vi "NanoScan ActiveX Sample.LV2018.vi"() -> ()   [LabVIEW 2018]
panel:
  in  "NanoScan.INanoScan":refnum<k7>
  out "Boolean":bool
  out "Sampling Res 1":sgl caption="Sampling Res" format="%.2f"
  out "Gain1":u32
  out "Aperture 1":cluster{"Intensity":sgl[], "Position":sgl[]}(graph)
  out "Sampling Res 2":sgl caption="Sampling Res" format="%.2f"
  out "Gain2":u32
  out "Aperture 2":cluster{"Intensity":sgl[], "Position":sgl[]}(graph)
  out "ROIs Aperture1":bool[](array[boolean])
  in  "Aperture":i32(slide) scale=1.0..2.0
  out "ROIs Aperture 2":bool[](array[boolean])
  in  "Position":sgl[](array[numeric]) format="%.2f"
  in  "Intensity":sgl[](array[numeric]) format="%.2f"
  in  "Ellipticity":sgl format="%.2f"
  in  "Roughness":sgl format="%.2f"
  in  "Goodness":sgl format="%.2f"
  in  "Irradiance":sgl format="%.2f"
  in  "Peak":sgl format="%.2f"
  in  "Centroid Pos":sgl format="%.2f"
  in  "BeamWidth":sgl format="%.2f"
  in  "Gain":i32
  in  "Set Gain":bool
  in  "Row":i32
  out "Parameters Array":string[][](array[string])
  in  "ROIs Ap2":i16
  in  "ROIs AP1":i16
  out "Intensity":sgl[](array[numeric]) format="%.2f"
  out "Position":sgl[](array[numeric]) format="%.2f"
  in  "Apr Right":sgl format="%.2f"
  in  "AprLeft":sgl format="%.2f"
  out "Parameters":i32[](listbox)
  in  "Filter":sgl=2.0 min=2 max=190 step=1 format="%.2f"
  in  "Set Filter":bool
  out "DAQ ON?":bool
  in  "Auto Find":bool
  in  "DAQ":bool caption="stop"
  in  "Exit":bool
  in  "13.5% Width":bool
  in  "Irradiance":bool
  in  "4Sigma Width":bool
  in  "Peak Pos":bool
  in  "50% Width":bool
  in  "Centroid Pos":bool
  in  "Peak Separation":bool caption="4Sigma Width 5"
  in  "Centroid Separation":bool
  in  "Gaussian Fit":bool
  in  "Ellipticity":bool
  in  "Select Sampling":sgl=0.09 min=0.0057 step=0.01 format="%.4f"
  in  "Set Sampling":bool
  out "Gains":u32[](array[numeric])
  in  "Select Rotation Rate":u16(ring) items=["1.25", "2.50", "5.00", "10.00", "20.00"]
  out "Measured Rotation [Hz]":sgl(knob) scale=1.25..20.0 scale format="%.2f"
  in  "Set Rotation":bool
  in  "Speed":sgl format="%.2f"
  in  "Gains 2":variant[](array[variant])
  out "pvarHeadInfo":variant
  in  "Speeds 2":variant[](array[variant])
  out "error out":errorcluster
  out "Speeds":sgl[](array[numeric]) format="%.2f"
  # "NanoScan"
  # "Parameters"
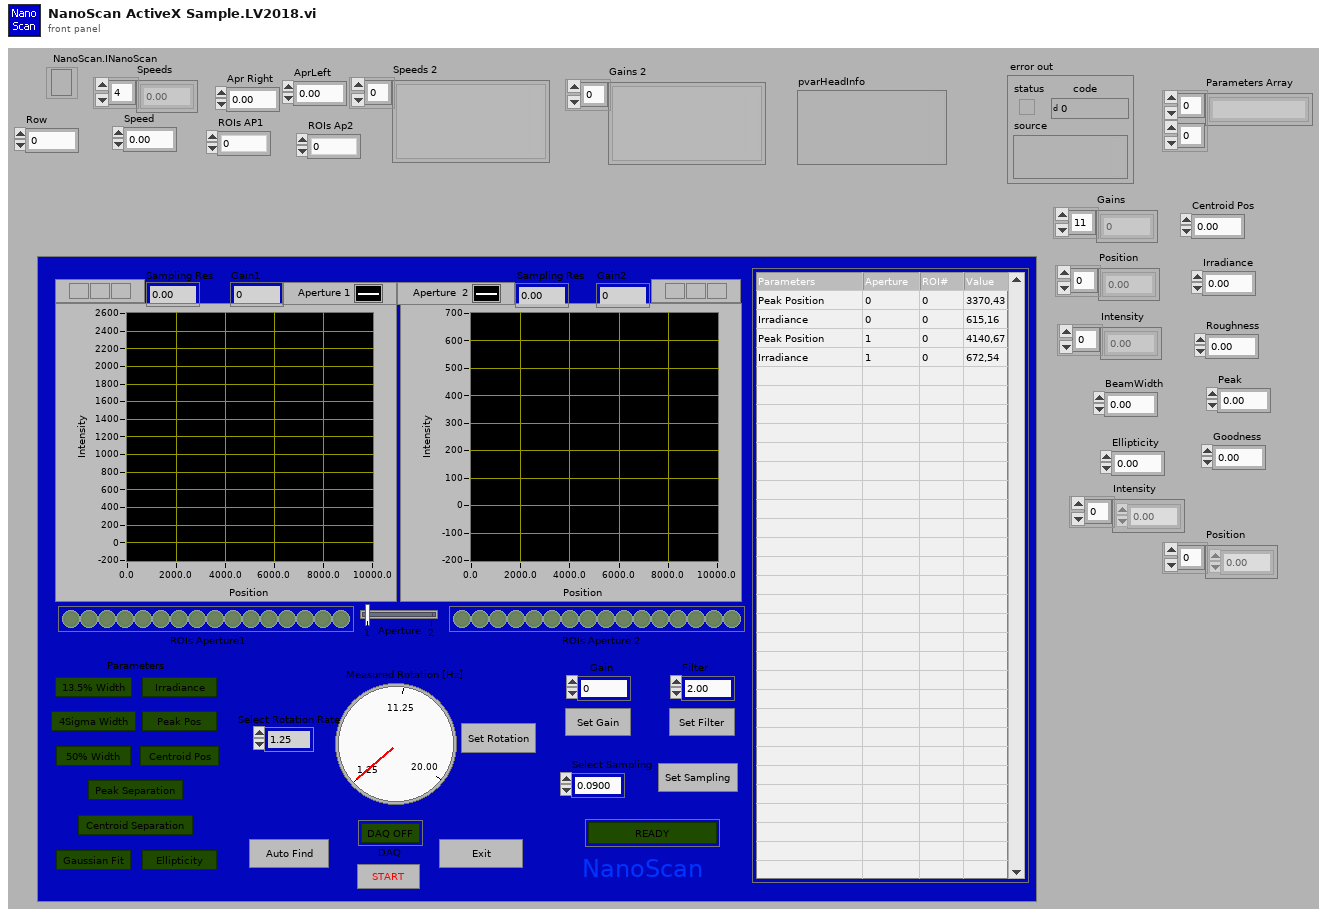
[diagram p1: front panel]
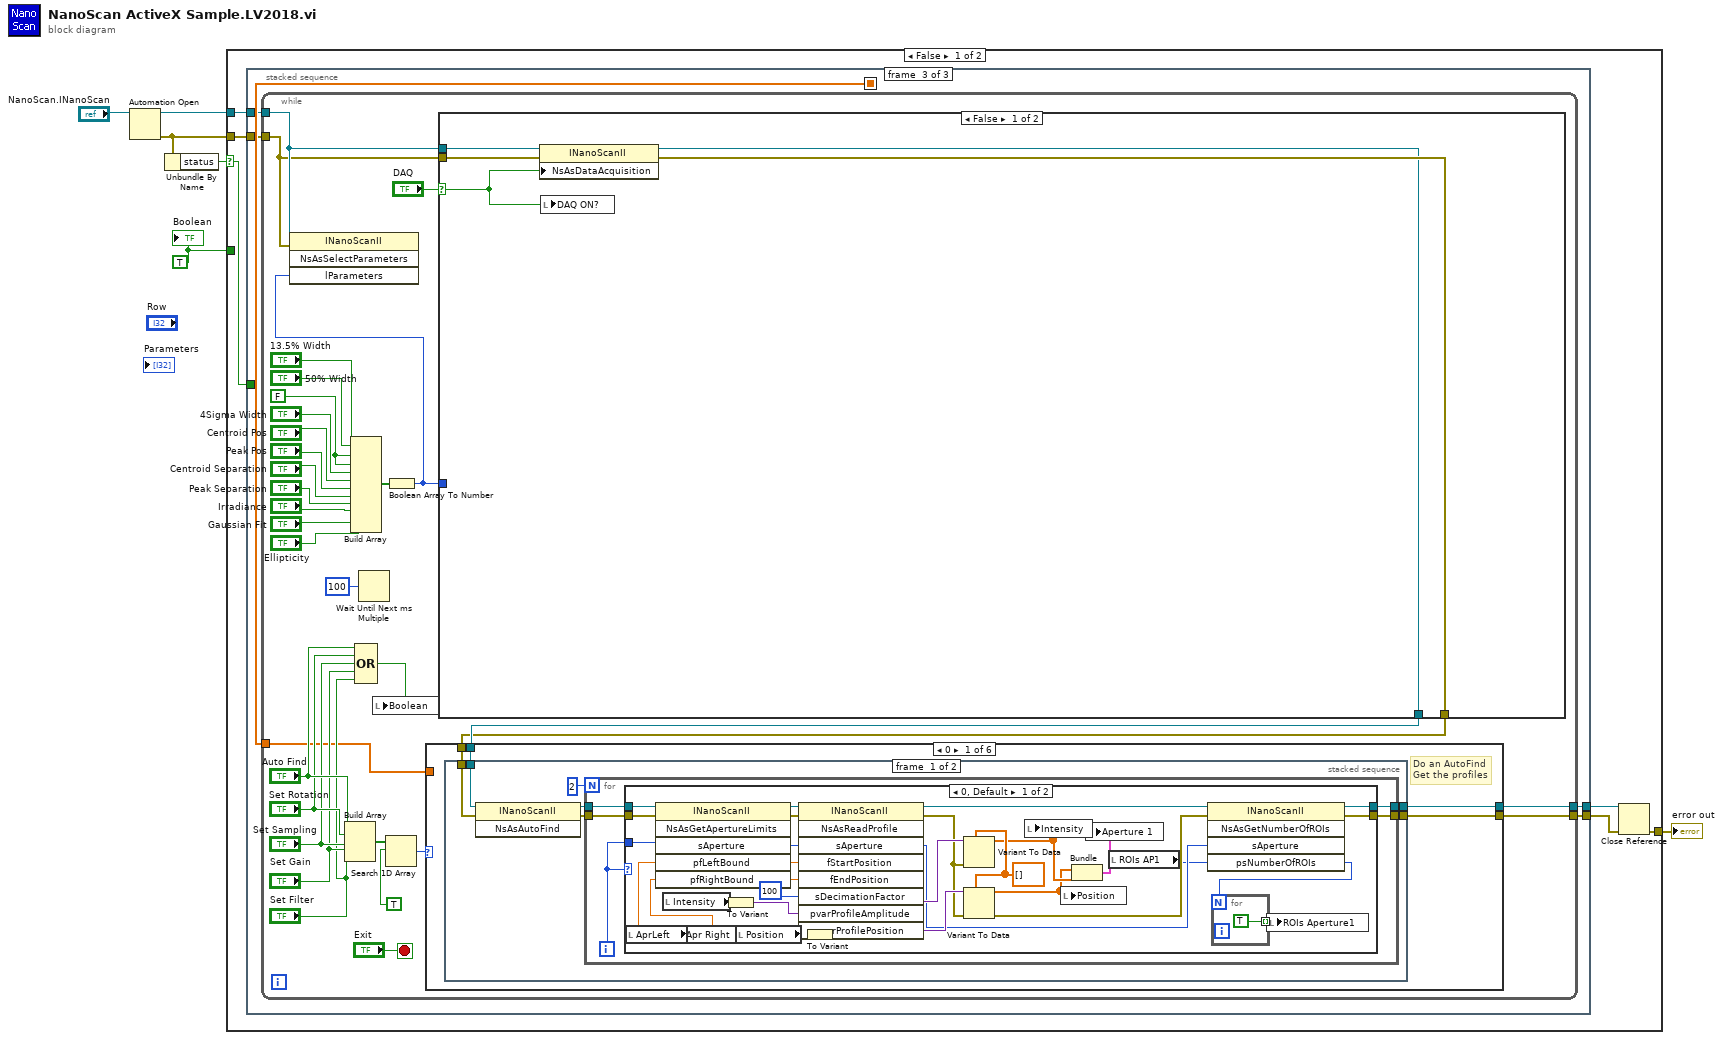
[diagram p0: block diagram]
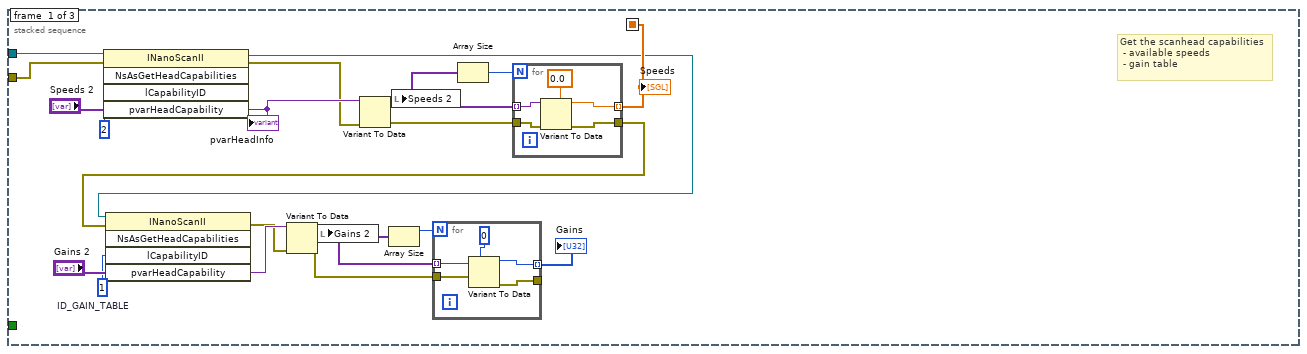
[diagram p2: hidden frame]
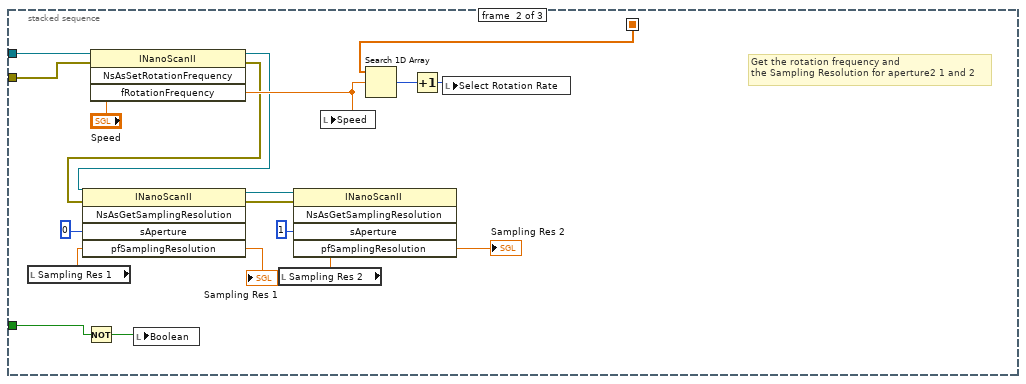
[diagram p3: hidden frame]
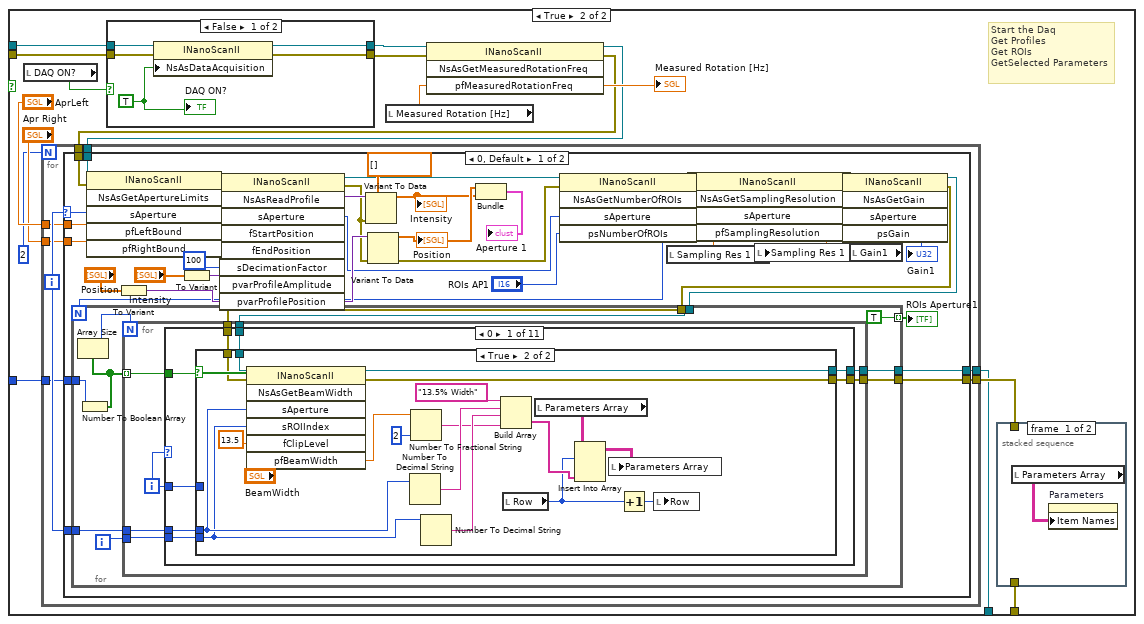
[diagram p4: hidden frame]
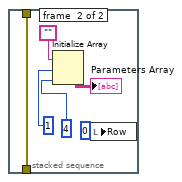
[diagram p5: hidden frame]
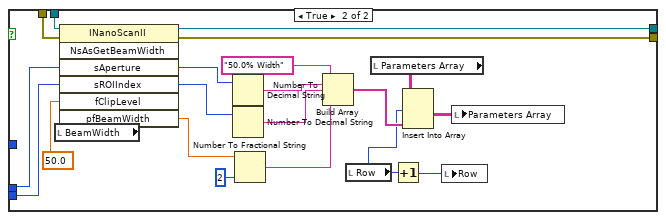
[diagram p8: hidden frame]
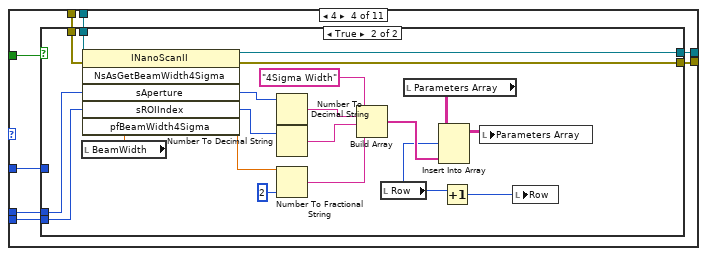
[diagram p10: hidden frame]
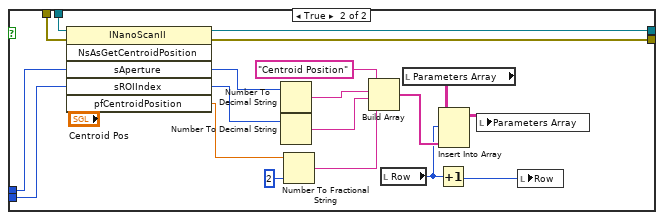
[diagram p13: hidden frame]
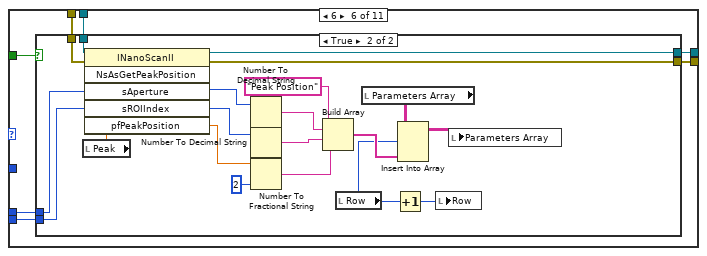
[diagram p14: hidden frame]
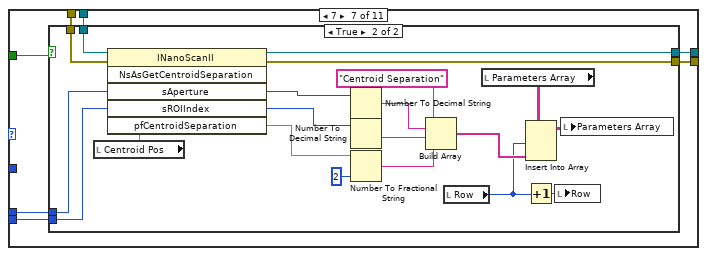
[diagram p16: hidden frame]
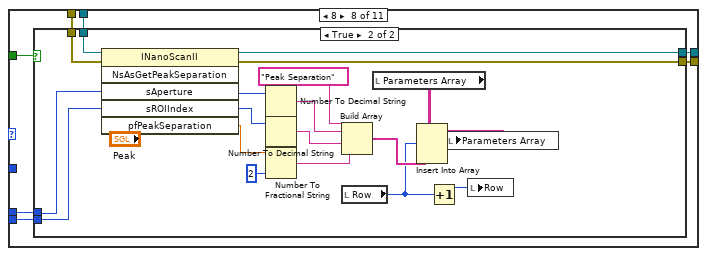
[diagram p18: hidden frame]
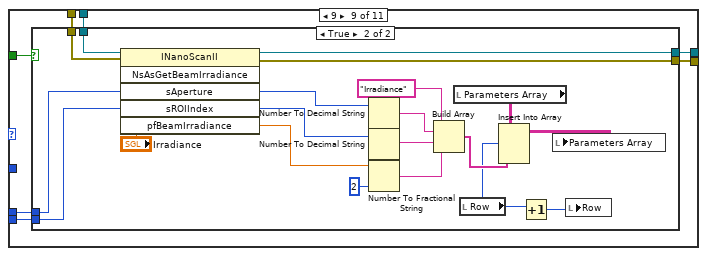
[diagram p20: hidden frame]
diagram:
  w1 = TRUE
  n1 = Automation Open(Automation Refnum="NanoScan.INanoScan") -> (Automation Refnum=w3:refnum<k7>, error out=w4:errorcluster)  [unwired: 1 in, 2 out]
  n2 = Unbundle By Name(w4) -> ("status"=w5:bool)
  n3 = case shown="False" w5 {
    selector: w5 -> [w12 w1002]
    tunnel: w4 -> [w11 w1000]
    tunnel: w3 -> [w10 w999]
    tunnel: [w7 w1000] -> w2
    tunnel: w1 -> [_ _]
    frame False {
      n4 = stacked-sequence {
        seq-local: [w27 _ _] -> [_ w61 w66]
        tunnel: w12 -> [_ w58 _]
        tunnel: w11 -> [w23 w43 w65]
        tunnel: w10 -> [w24 w56 w64]
        tunnel: [_ _ w63] -> w9
        tunnel: [_ _ w62] -> w8
        frame #0 {
          w17 = 1  # ID_GAIN_TABLE
          # "Get the scanhead capabilities\n - available speeds\n - gain table"
          n5 = invoke class="INanoScanII" method="NsAsGetHeadCapabilities"(reference=w24, error in=w23, "lCapabilityID"=2, "pvarHeadCapability"="Speeds 2") -> (reference out=w16:refnum<k7>, error out=w19:errorcluster, "pvarHeadCapability"=w22:variant)  [unwired: 1 in, 2 out]
          "pvarHeadInfo" <- w22
          n6 = Variant To Data(error in=w19, Variant=w22) -> (data=w26:variant[], error out=w28:errorcluster)  [unwired: 1 in]
          n7 = local write "Speeds 2"(w26) -> ()
          n8 = Array Size(array=w26) -> (size(s)=w25:i32)
          n9 = for {
            N: w25 -> [_]
            tunnel: w26 -> [w37] mode=indexing
            tunnel: [w36] -> w27 mode=indexing
            tunnel: w28 -> [w35]
            tunnel: [w33] -> w15
            n10 = Variant To Data(error in=w35, type=sgl 0.0, Variant=w37) -> (data=w36:sgl, error out=w33:errorcluster)
          }
          "Speeds" <- w27
          n11 = invoke class="INanoScanII" method="NsAsGetHeadCapabilities"(reference=w16, error in=w15, "lCapabilityID"=w17, "pvarHeadCapability"="Gains 2") -> (error out=w13:errorcluster, "pvarHeadCapability"=w14:variant)  [unwired: 1 in, 3 out]
          n12 = Variant To Data(error in=w13, Variant=w14) -> (data=w29:variant[], error out=w30:errorcluster)  [unwired: 1 in]
          n13 = local write "Gains 2"(w29) -> ()
          n14 = Array Size(array=w29) -> (size(s)=w31:i32)
          n15 = for {
            N: w31 -> [_]
            tunnel: w29 -> [w41] mode=indexing
            tunnel: w30 -> [w40]
            tunnel: [w39] -> w32 mode=indexing
            tunnel: [w38] -> _
            n16 = Variant To Data(error in=w40, type=u32 0, Variant=w41) -> (data=w39:u32, error out=w38:errorcluster)
          }
          "Gains" <- w32
        }
        frame #1 {
          # "Get the rotation frequency and\nthe Sampling Resolution for aperture2 1 and 2"
          n17 = local read "Sampling Res 1"() -> (w46:sgl)
          n18 = Not(x=w58) -> (.not. x?=w57:bool)
          n19 = invoke class="INanoScanII" method="NsAsSetRotationFrequency"(reference=w56, error in=w43, "fRotationFrequency"="Speed") -> (reference out=w53:refnum<k7>, error out=w52:errorcluster, "fRotationFrequency"=w55:sgl)  [unwired: 1 in, 1 out]
          n20 = invoke class="INanoScanII" method="NsAsGetSamplingResolution"(reference=w53, error in=w52, "sAperture"=i16 0, "pfSamplingResolution"=w46) -> (reference out=w50:refnum<k7>, error out=w49:errorcluster, "pfSamplingResolution"=→"Sampling Res 1":sgl)  [unwired: 1 in, 2 out]
          n21 = local write "Boolean"(w57) -> ()
          n22 = local read "Sampling Res 2"() -> (w48:sgl)
          n23 = invoke class="INanoScanII" method="NsAsGetSamplingResolution"(reference=w50, error in=w49, "sAperture"=i16 1, "pfSamplingResolution"=w48) -> ("pfSamplingResolution"=→"Sampling Res 2":sgl)  [unwired: 1 in, 4 out]
          n24 = local write "Speed"(w55) -> ()
          n25 = Search 1D Array(1D array=w61, element=w55) -> (index of element=w60:i32)  [unwired: 1 out]
          n26 = Increment(x=w60) -> (x+1=w59:i32)
          n27 = local write "Select Rotation Rate"(w59) -> ()
        }
        frame #2 {
          n28 = while {
            tunnel: w66 -> [w72]
            tunnel: w65 -> [w73]
            tunnel: w64 -> [w74]
            tunnel: [w69] -> w63
            tunnel: [w68] -> w62
            stop <- "Exit" stop-if-true
            w91 = FALSE
            n29 = Build Array("Auto Find", "Set Rotation", "Set Sampling", "Set Gain", "Set Filter") -> (w97:bool[])
            n30 = Build Array("13.5% Width", "50% Width", w91, w91, "4Sigma Width", "Centroid Pos", "Peak Pos", "Centroid Separation", "Peak Separation", "Irradiance", "Gaussian Fit", "Ellipticity") -> (w82:bool[])
            n31 = Compound Arithmetic op=OR("Auto Find", "Set Rotation", "Set Sampling", "Set Gain", "Set Filter") -> (w76:bool)
            n32 = Wait Until Next ms Multiple(millisecond multiple=u32 100) -> ()  [unwired: 1 out]
            n33 = local write "Boolean"(w76) -> ()
            n34 = Search 1D Array(1D array=w97, element=TRUE) -> (index of element=w95:i32)  [unwired: 1 out]
            n35 = Boolean Array To Number(Boolean array=w82) -> (number=w67:u32)
            n36 = invoke class="INanoScanII" method="NsAsSelectParameters"(reference=w74, error in=w73, "lParameters"=w67) -> ()  [unwired: 1 in, 4 out]
            n37 = case shown="False" "DAQ" {
              selector: "DAQ" -> [w99 _]
              tunnel: w67 -> [_ w115]
              tunnel: w74 -> [w103 w114]
              tunnel: w73 -> [w102 w113]
              tunnel: [w100 w105] -> w71
              tunnel: [w101 w104] -> w70
              frame False {
                n38 = property class="INanoScanII"(reference=w103, error in=w102, "NsAsDataAcquisition"=w99) -> (reference out=w100:refnum<k7>, error out=w101:errorcluster)
                n39 = local write "DAQ ON?"(w99) -> ()
              }
              frame True {
                # "Start the Daq\nGet Profiles\nGet ROIs\nGetSelected Parameters"
                n40 = local read "DAQ ON?"() -> (w119:bool)
                n41 = case shown="False" w119 {
                  tunnel: w114 -> [w866 w868]
                  tunnel: w113 -> [w864 w867]
                  tunnel: [w865 w868] -> w112
                  tunnel: [w863 w867] -> w111
                  frame False {
                    w862 = TRUE ("NsAsDataAcquisition")
                    n42 = property class="INanoScanII"(reference=w866, error in=w864, "NsAsDataAcquisition"=w862) -> (reference out=w865:refnum<k7>, error out=w863:errorcluster)
                    "DAQ ON?" <- w862
                  }
                  frame True {
                  }
                }
                n43 = local read "Measured Rotation [Hz]"() -> (w110:sgl)
                n44 = invoke class="INanoScanII" method="NsAsGetMeasuredRotationFreq"(reference=w112, error in=w111, "pfMeasuredRotationFreq"=w110) -> (reference out=w108:refnum<k7>, error out=w107:errorcluster, "pfMeasuredRotationFreq"=→"Measured Rotation [Hz]":sgl)  [unwired: 1 in, 1 out]
                n45 = for {
                  N: i16 2 ("sAperture") -> [_]
                  tunnel: "AprLeft" -> [w133]
                  tunnel: "Apr Right" -> [w132]
                  tunnel: w115 -> [w131]
                  tunnel: w108 -> [w130]
                  tunnel: w107 -> [w129]
                  tunnel: [w128] -> w105
                  tunnel: [w127] -> w106
                  i -> [w134]
                  n46 = case shown="0, Default" w134 {
                    selector: w134 -> [w166 w535]
                    tunnel: w133 -> [w168 w537]
                    tunnel: w132 -> [w167 w536]
                    tunnel: w131 -> [w178 w541]
                    tunnel: w134 -> [w177 w540]
                    tunnel: w130 -> [w170 w539]
                    tunnel: w129 -> [w169 w538]
                    tunnel: [w138 w509] -> w128
                    tunnel: [w137 w508] -> w127
                    frame 0, Default {
                      n47 = invoke class="INanoScanII" method="NsAsGetApertureLimits"(reference=w170, error in=w169, "sAperture"=w166, "pfLeftBound"=w168, "pfRightBound"=w167) -> (reference out=w165:refnum<k7>, error out=w164:errorcluster, "sAperture"=w163:i16, "pfLeftBound"=w159:sgl, "pfRightBound"=w158:sgl)  [unwired: 1 in, 1 out]
                      n48 = To Variant(anything="Position") -> (Variant=w160:variant)
                      n49 = To Variant(anything="Intensity") -> (Variant=w162:variant)
                      n50 = invoke class="INanoScanII" method="NsAsReadProfile"(reference=w165, error in=w164, "sAperture"=w163, "fStartPosition"=w159, "fEndPosition"=w158, "sDecimationFactor"=i16 100, "pvarProfileAmplitude"=w162, "pvarProfilePosition"=w160) -> (reference out=w154:refnum<k7>, error out=w155:errorcluster, "sAperture"=w152:i16, "pvarProfileAmplitude"=w157:variant, "pvarProfilePosition"=w156:variant)  [unwired: 1 in, 4 out]
                      n51 = Variant To Data(error in=w155, type=sgl[] [] ("Intensity"), Variant=w157) -> (data=w171:sgl[])  [unwired: 1 out]
                      "Intensity" <- w171
                      n52 = Variant To Data(error in=w155, Variant=w156) -> (data=w172:sgl[], error out=w153:errorcluster)  [unwired: 1 in]
                      "Position" <- w172
                      n53 = Bundle("Position"=w172, "Intensity"=w171) -> (→"Aperture 1":cluster{"Position":sgl[], "Intensity":sgl[]})  [unwired: 1 out]
                      n54 = invoke class="INanoScanII" method="NsAsGetNumberOfROIs"(reference=w154, error in=w153, "sAperture"=w152, "psNumberOfROIs"="ROIs AP1") -> (reference out=w150:refnum<k7>, error out=w149:errorcluster, "sAperture"=w148:i16, "psNumberOfROIs"=w142:i16)  [unwired: 1 in, 1 out]
                      n55 = local read "Sampling Res 1"() -> (w143:sgl)
                      n56 = invoke class="INanoScanII" method="NsAsGetSamplingResolution"(reference=w150, error in=w149, "sAperture"=w148, "pfSamplingResolution"=w143) -> (reference out=w147:refnum<k7>, error out=w146:errorcluster, "sAperture"=w145:i16, "pfSamplingResolution"=w144:sgl)  [unwired: 1 in, 1 out]
                      n57 = local write "Sampling Res 1"(w144) -> ()
                      n58 = local read "Gain1"() -> (w136:u32)
                      n59 = invoke class="INanoScanII" method="NsAsGetGain"(reference=w147, error in=w146, "sAperture"=w145, "psGain"=w136) -> (reference out=w139:refnum<k7>, error out=w140:errorcluster, "psGain"=→"Gain1":i16)  [unwired: 1 in, 2 out]
                      n60 = for {
                        N: w142 -> [_]
                        tunnel: w178 -> [w188]
                        tunnel: w177 -> [w185]
                        tunnel: [TRUE] -> w141 mode=indexing
                        tunnel: w140 -> [w183]
                        tunnel: w139 -> [w182]
                        tunnel: [w181] -> w138
                        tunnel: [w180] -> w137
                        i -> [w179]
                        n61 = Number To Boolean Array(number=w188) -> (Boolean array=w186:bool[])
                        n62 = Array Size(array=w186) -> (size(s)=w187:i32)
                        n63 = for {
                          N: w187 -> [_]
                          tunnel: w186 -> [w193] mode=indexing
                          tunnel: w185 -> [w196]
                          tunnel: w179 -> [w195]
                          tunnel: w183 -> [w192]
                          tunnel: w182 -> [w191]
                          tunnel: [w190] -> w181
                          tunnel: [w189] -> w180
                          i -> [w194]
                          n64 = case shown="0" w194 {
                            tunnel: w193 -> [w204 w233 _ w264 w295 w324 w353 w380 w411 w440 w477]
                            tunnel: w196 -> [w203 w231 _ w265 w291 w323 w352 w382 w410 w439 w476]
                            tunnel: w195 -> [w202 w226 _ w263 w290 w322 w351 w381 w409 w438 w475]
                            tunnel: w194 -> [w201 w232 _ w266 _ _ _ _ _ _ _]
                            tunnel: w192 -> [w200 w229 w257 w261 w289 w319 w349 w378 w407 w434 w471]
                            tunnel: w191 -> [w199 w230 w258 w262 w294 w318 w350 w379 w408 w435 w472]
                            tunnel: [w198 w227 w258 w260 w293 w321 w348 w377 w406 w437 w474] -> w190
                            tunnel: [w197 w228 w257 w259 w292 w320 w347 w376 w405 w436 w473] -> w189
                            frame 0 {
                              n65 = case shown="True" w204 {
                                tunnel: w203 -> [_ w210]
                                tunnel: w202 -> [_ w209]
                                tunnel: w201 -> [_ _]
                                tunnel: w200 -> [w205 w215]
                                tunnel: w199 -> [w206 w214]
                                tunnel: [w206 w213] -> w198
                                tunnel: [w205 w212] -> w197
                                frame False {
                                }
                                frame True {
                                n66 = invoke class="INanoScanII" method="NsAsGetBeamWidth"(reference=w214, error in=w215, "sAperture"=w210, "sROIIndex"=w209, "fClipLevel"=13.5, "pfBeamWidth"="BeamWidth") -> (reference out=w213:refnum<k7>, error out=w212:errorcluster, "pfBeamWidth"=w207:sgl)  [unwired: 1 in, 4 out]
                                n67 = Number To Decimal String(number=w210) -> (decimal integer string=w224:string)  [unwired: 1 out]
                                n68 = Number To Fractional String(number=w207, precision (6)=i16 2) -> (F-format string=w222:string)  [unwired: 2 out]
                                n69 = Number To Decimal String(number=w209) -> (decimal integer string=w223:string)  [unwired: 1 out]
                                n70 = Build Array("13.5% Width", w224, w223, w222) -> (w221:string[])
                                n71 = local read "Row"() -> (w217:i32)
                                n72 = local read "Parameters Array"() -> (w219:string[][])
                                n73 = Insert Into Array(array=w219, index (row)=w217, new element=w221) -> (w218:string[][])  [unwired: 1 in]
                                n74 = local write "Parameters Array"(w218) -> ()
                                n75 = Increment(x=w217) -> (x+1=w220:i32)
                                n76 = local write "Row"(w220) -> ()
                                }
                              }
                            }
                            frame 1 {
                              n77 = case shown="False" w233 {
                                tunnel: w232 -> [_ _]
                                tunnel: w231 -> [_ w244]
                                tunnel: w230 -> [w234 w246]
                                tunnel: w229 -> [w235 w245]
                                tunnel: [w235 w236] -> w228
                                tunnel: [w234 w238] -> w227
                                tunnel: w226 -> [_ w243]
                                frame False {
                                }
                                frame True {
                                n78 = local read "BeamWidth"() -> (w241:sgl)
                                n79 = invoke class="INanoScanII" method="NsAsGetBeamWidth"(reference=w246, error in=w245, "sAperture"=w244, "sROIIndex"=w243, "fClipLevel"=sgl 50.0, "pfBeamWidth"=w241) -> (reference out=w238:refnum<k7>, error out=w236:errorcluster, "sAperture"=w237:i16, "sROIIndex"=w240:i16, "pfBeamWidth"=w239:sgl)  [unwired: 1 in, 2 out]
                                n80 = Number To Decimal String(number=w237) -> (decimal integer string=w255:string)  [unwired: 1 out]
                                n81 = Number To Decimal String(number=w240) -> (decimal integer string=w254:string)  [unwired: 1 out]
                                n82 = Number To Fractional String(number=w239, precision (6)=i16 2) -> (F-format string=w253:string)  [unwired: 2 out]
                                n83 = Build Array("50.0% Width", w255, w254, w253) -> (w251:string[])
                                n84 = local read "Row"() -> (w249:i32)
                                n85 = local read "Parameters Array"() -> (w252:string[][])
                                n86 = Increment(x=w249) -> (x+1=w248:i32)
                                n87 = Insert Into Array(array=w252, index (row)=w249, new element=w251) -> (w250:string[][])  [unwired: 1 in]
                                n88 = local write "Row"(w248) -> ()
                                n89 = local write "Parameters Array"(w250) -> ()
                                }
                              }
                            }
                            frame Default {
                            }
                            frame 4 {
                              n90 = case shown="True" w264 {
                                tunnel: w266 -> [_ _]
                                tunnel: w265 -> [_ w273]
                                tunnel: w263 -> [_ w272]
                                tunnel: w262 -> [w268 w278]
                                tunnel: w261 -> [w267 w277]
                                tunnel: [w268 w276] -> w260
                                tunnel: [w267 w275] -> w259
                                frame False {
                                }
                                frame True {
                                n91 = local read "BeamWidth"() -> (w274:sgl)
                                n92 = invoke class="INanoScanII" method="NsAsGetBeamWidth4Sigma"(reference=w278, error in=w277, "sAperture"=w273, "sROIIndex"=w272, "pfBeamWidth4Sigma"=w274) -> (reference out=w276:refnum<k7>, error out=w275:errorcluster, "sAperture"=w271:i16, "sROIIndex"=w270:i16, "pfBeamWidth4Sigma"=w269:sgl)  [unwired: 1 in, 1 out]
                                n93 = Number To Decimal String(number=w271) -> (decimal integer string=w287:string)  [unwired: 1 out]
                                n94 = Number To Decimal String(number=w270) -> (decimal integer string=w286:string)  [unwired: 1 out]
                                n95 = Number To Fractional String(number=w269, precision (6)=i16 2) -> (F-format string=w285:string)  [unwired: 2 out]
                                n96 = Build Array("4Sigma Width", w287, w286, w285) -> (w284:string[])
                                n97 = local read "Row"() -> (w281:i32)
                                n98 = local read "Parameters Array"() -> (w282:string[][])
                                n99 = Insert Into Array(array=w282, index (row)=w281, new element=w284) -> (w283:string[][])  [unwired: 1 in]
                                n100 = Increment(x=w281) -> (x+1=w280:i32)
                                n101 = local write "Parameters Array"(w283) -> ()
                                n102 = local write "Row"(w280) -> ()
                                }
                              }
                            }
                            frame 5 {
                              n103 = case shown="False" w295 {
                                tunnel: w294 -> [w296 w307]
                                tunnel: [w296 w306] -> w293
                                tunnel: [w297 w305] -> w292
                                tunnel: w291 -> [_ w303]
                                tunnel: w290 -> [_ w302]
                                tunnel: w289 -> [w297 w298]
                                frame False {
                                }
                                frame True {
                                n104 = invoke class="INanoScanII" method="NsAsGetCentroidPosition"(reference=w307, error in=w298, "sAperture"=w303, "sROIIndex"=w302, "pfCentroidPosition"="Centroid Pos") -> (reference out=w306:refnum<k7>, error out=w305:errorcluster, "sAperture"=w301:i16, "sROIIndex"=w300:i16, "pfCentroidPosition"=w299:sgl)  [unwired: 1 in, 1 out]
                                n105 = Number To Decimal String(number=w301) -> (decimal integer string=w316:string)  [unwired: 1 out]
                                n106 = Number To Decimal String(number=w300) -> (decimal integer string=w315:string)  [unwired: 1 out]
                                n107 = Number To Fractional String(number=w299, precision (6)=i16 2) -> (F-format string=w314:string)  [unwired: 2 out]
                                n108 = Build Array("Centroid Position", w316, w315, w314) -> (w313:string[])
                                n109 = local read "Row"() -> (w309:i32)
                                n110 = local read "Parameters Array"() -> (w312:string[][])
                                n111 = Increment(x=w309) -> (x+1=w310:i32)
                                n112 = Insert Into Array(array=w312, index (row)=w309, new element=w313) -> (w311:string[][])  [unwired: 1 in]
                                n113 = local write "Parameters Array"(w311) -> ()
                                n114 = local write "Row"(w310) -> ()
                                }
                              }
                            }
                            frame 6 {
                              n115 = case shown="True" w324 {
                                tunnel: w323 -> [_ w331]
                                tunnel: w322 -> [_ w330]
                                tunnel: [w326 w336] -> w321
                                tunnel: [w325 w335] -> w320
                                tunnel: w319 -> [w325 w334]
                                tunnel: w318 -> [w326 w333]
                                frame False {
                                }
                                frame True {
                                n116 = local read "Peak"() -> (w332:sgl)
                                n117 = invoke class="INanoScanII" method="NsAsGetPeakPosition"(reference=w333, error in=w334, "sAperture"=w331, "sROIIndex"=w330, "pfPeakPosition"=w332) -> (reference out=w336:refnum<k7>, error out=w335:errorcluster, "sAperture"=w329:i16, "sROIIndex"=w328:i16, "pfPeakPosition"=w327:sgl)  [unwired: 1 in, 1 out]
                                n118 = Number To Decimal String(number=w329) -> (decimal integer string=w345:string)  [unwired: 1 out]
                                n119 = Number To Decimal String(number=w328) -> (decimal integer string=w344:string)  [unwired: 1 out]
                                n120 = Number To Fractional String(number=w327, precision (6)=i16 2) -> (F-format string=w343:string)  [unwired: 2 out]
                                n121 = Build Array("Peak Position", w345, w344, w343) -> (w342:string[])
                                n122 = local read "Row"() -> (w339:i32)
                                n123 = local read "Parameters Array"() -> (w340:string[][])
                                n124 = Increment(x=w339) -> (x+1=w338:i32)
                                n125 = Insert Into Array(array=w340, index (row)=w339, new element=w342) -> (w341:string[][])  [unwired: 1 in]
                                n126 = local write "Row"(w338) -> ()
                                n127 = local write "Parameters Array"(w341) -> ()
                                }
                              }
                            }
                            frame 7 {
                              n128 = case shown="True" w353 {
                                tunnel: w352 -> [_ w362]
                                tunnel: w351 -> [_ w361]
                                tunnel: w350 -> [w355 w364]
                                tunnel: w349 -> [w354 w363]
                                tunnel: [w355 w360] -> w348
                                tunnel: [w354 w359] -> w347
                                frame False {
                                }
                                frame True {
                                n129 = local read "Centroid Pos"() -> (w365:sgl)
                                n130 = invoke class="INanoScanII" method="NsAsGetCentroidSeparation"(reference=w364, error in=w363, "sAperture"=w362, "sROIIndex"=w361, "pfCentroidSeparation"=w365) -> (reference out=w360:refnum<k7>, error out=w359:errorcluster, "sAperture"=w358:i16, "sROIIndex"=w357:i16, "pfCentroidSeparation"=w356:sgl)  [unwired: 1 in, 1 out]
                                n131 = Number To Decimal String(number=w358) -> (decimal integer string=w374:string)  [unwired: 1 out]
                                n132 = Number To Decimal String(number=w357) -> (decimal integer string=w373:string)  [unwired: 1 out]
                                n133 = Number To Fractional String(number=w356, precision (6)=i16 2) -> (F-format string=w372:string)  [unwired: 2 out]
                                n134 = Build Array("Centroid Separation", w374, w373, w372) -> (w369:string[])
                                n135 = local read "Row"() -> (w368:i32)
                                n136 = local read "Parameters Array"() -> (w371:string[][])
                                n137 = Insert Into Array(array=w371, index (row)=w368, new element=w369) -> (w370:string[][])  [unwired: 1 in]
                                n138 = Increment(x=w368) -> (x+1=w367:i32)
                                n139 = local write "Row"(w367) -> ()
                                n140 = local write "Parameters Array"(w370) -> ()
                                }
                              }
                            }
                            frame 8 {
                              n141 = case shown="True" w380 {
                                tunnel: w382 -> [_ w386]
                                tunnel: w381 -> [_ w385]
                                tunnel: w379 -> [w384 w394]
                                tunnel: w378 -> [w383 w393]
                                tunnel: [w384 w392] -> w377
                                tunnel: [w383 w391] -> w376
                                frame False {
                                }
                                frame True {
                                n142 = invoke class="INanoScanII" method="NsAsGetPeakSeparation"(reference=w394, error in=w393, "sAperture"=w386, "sROIIndex"=w385, "pfPeakSeparation"="Peak") -> (reference out=w392:refnum<k7>, error out=w391:errorcluster, "sAperture"=w390:i16, "sROIIndex"=w389:i16, "pfPeakSeparation"=w388:sgl)  [unwired: 1 in, 1 out]
                                n143 = Number To Decimal String(number=w390) -> (decimal integer string=w403:string)  [unwired: 1 out]
                                n144 = Number To Decimal String(number=w389) -> (decimal integer string=w402:string)  [unwired: 1 out]
                                n145 = Number To Fractional String(number=w388, precision (6)=i16 2) -> (F-format string=w401:string)  [unwired: 2 out]
                                n146 = Build Array("Peak Separation", w403, w402, w401) -> (w398:string[])
                                n147 = local read "Row"() -> (w397:i32)
                                n148 = local read "Parameters Array"() -> (w400:string[][])
                                n149 = Insert Into Array(array=w400, index (row)=w397, new element=w398) -> (w399:string[][])  [unwired: 1 in]
                                n150 = Increment(x=w397) -> (x+1=w396:i32)
                                n151 = local write "Parameters Array"(w399) -> ()
                                n152 = local write "Row"(w396) -> ()
                                }
                              }
                            }
                            frame 9 {
                              n153 = case shown="True" w411 {
                                tunnel: w410 -> [_ w419]
                                tunnel: w409 -> [_ w418]
                                tunnel: w408 -> [w413 w423]
                                tunnel: w407 -> [w412 w422]
                                tunnel: [w413 w421] -> w406
                                tunnel: [w412 w414] -> w405
                                frame False {
                                }
                                frame True {
                                n154 = invoke class="INanoScanII" method="NsAsGetBeamIrradiance"(reference=w423, error in=w422, "sAperture"=w419, "sROIIndex"=w418, "pfBeamIrradiance"="Irradiance") -> (reference out=w421:refnum<k7>, error out=w414:errorcluster, "sAperture"=w417:i16, "sROIIndex"=w416:i16, "pfBeamIrradiance"=w415:sgl)  [unwired: 1 in, 1 out]
                                n155 = Number To Decimal String(number=w417) -> (decimal integer string=w432:string)  [unwired: 1 out]
                                n156 = Number To Decimal String(number=w416) -> (decimal integer string=w431:string)  [unwired: 1 out]
                                n157 = Number To Fractional String(number=w415, precision (6)=i16 2) -> (F-format string=w430:string)  [unwired: 2 out]
                                n158 = Build Array("Irradiance", w432, w431, w430) -> (w427:string[])
                                n159 = local read "Parameters Array"() -> (w429:string[][])
                                n160 = local read "Row"() -> (w426:i32)
                                n161 = Insert Into Array(array=w429, index (row)=w426, new element=w427) -> (w428:string[][])  [unwired: 1 in]
                                n162 = Increment(x=w426) -> (x+1=w425:i32)
                                n163 = local write "Parameters Array"(w428) -> ()
                                n164 = local write "Row"(w425) -> ()
                                }
                              }
                            }
                            frame 10 {
                              n165 = case shown="True" w440 {
                                tunnel: w439 -> [_ w452]
                                tunnel: w438 -> [_ w451]
                                tunnel: [w442 w454] -> w437
                                tunnel: [w441 w453] -> w436
                                tunnel: w435 -> [w442 w444]
                                tunnel: w434 -> [w441 w443]
                                frame False {
                                }
                                frame True {
                                n166 = invoke class="INanoScanII" method="NsAsGetGaussianFit"(reference=w444, error in=w443, "sAperture"=w452, "sROIIndex"=w451, "pfGoodnessFit"="Goodness", "pfRoughnessFit"="Roughness") -> (reference out=w454:refnum<k7>, error out=w453:errorcluster, "sAperture"=w448:i16, "sROIIndex"=w447:i16, "pfGoodnessFit"=w446:sgl, "pfRoughnessFit"=w445:sgl)  [unwired: 1 in, 1 out]
                                n167 = Number To Decimal String(number=w448) -> (decimal integer string=w467:string)  [unwired: 1 out]
                                n168 = Number To Decimal String(number=w447) -> (decimal integer string=w466:string)  [unwired: 1 out]
                                n169 = Number To Fractional String(number=w446, precision (6)=i16 2) -> (F-format string=w469:string)  [unwired: 2 out]
                                n170 = Number To Fractional String(number=w445, precision (6)=i16 2) -> (F-format string=w465:string)  [unwired: 2 out]
                                n171 = local read "Row"() -> (w460:i32)
                                n172 = Build Array("Goodness of Fit", w467, w466, w469) -> (w464:string[])
                                n173 = Build Array("Roughness of Fit", w467, w466, w465) -> (w463:string[])
                                n174 = local read "Parameters Array"() -> (w457:string[][])
                                n175 = Insert Into Array(array=w457, index (row)=w460, new element=w464) -> (w462:string[][])  [unwired: 1 in]
                                n176 = Increment(x=w460) -> (x+1=w459:i32)
                                n177 = local write "Parameters Array"(w462) -> ()
                                n178 = Insert Into Array(array=w462, index (row)=w459, new element=w463) -> (w461:string[][])  [unwired: 1 in]
                                n179 = Increment(x=w459) -> (x+1=w458:i32)
                                n180 = local write "Parameters Array"(w461) -> ()
                                n181 = local write "Row"(w458) -> ()
                                }
                              }
                            }
                            frame 11 {
                              n182 = case shown="True" w477 {
                                tunnel: w476 -> [_ _]
                                tunnel: w475 -> [_ w483]
                                tunnel: [w479 w487] -> w474
                                tunnel: [w478 w486] -> w473
                                tunnel: w472 -> [w479 w485]
                                tunnel: w471 -> [w478 w484]
                                frame False {
                                }
                                frame True {
                                n183 = invoke class="INanoScanII" method="NsAsGetBeamEllipticity"(reference=w485, error in=w484, "sROIIndex"=w483, "pfBeamEllipticity"="Ellipticity") -> (reference out=w487:refnum<k7>, error out=w486:errorcluster, "sROIIndex"=w481:i16, "pfBeamEllipticity"=w480:sgl)  [unwired: 1 in, 1 out]
                                n184 = Number To Decimal String(number=w481) -> (decimal integer string=w495:string)  [unwired: 1 out]
                                n185 = Number To Fractional String(number=w480, precision (6)=i16 2) -> (F-format string=w494:string)  [unwired: 2 out]
                                n186 = Build Array("Ellipticity", "", w495, w494) -> (w491:string[])
                                n187 = local read "Row"() -> (w490:i32)
                                n188 = local read "Parameters Array"() -> (w493:string[][])
                                n189 = Insert Into Array(array=w493, index (row)=w490, new element=w491) -> (w492:string[][])  [unwired: 1 in]
                                n190 = Increment(x=w490) -> (x+1=w489:i32)
                                n191 = local write "Parameters Array"(w492) -> ()
                                n192 = local write "Row"(w489) -> ()
                                }
                              }
                            }
                          }
                        }
                      }
                      "ROIs Aperture1" <- w141
                    }
                    frame 1 {
                      w503 = sgl[] [] ("Intensity")
                      n193 = local read "Position"() -> (w504:sgl[])
                      n194 = invoke class="INanoScanII" method="NsAsGetApertureLimits"(reference=w539, error in=w538, "sAperture"=w535, "pfLeftBound"=w537, "pfRightBound"=w536) -> (reference out=w534:refnum<k7>, error out=w533:errorcluster, "sAperture"=w532:i16, "pfLeftBound"=w528:sgl, "pfRightBound"=w527:sgl)  [unwired: 1 in, 1 out]
                      n195 = local read "Intensity"() -> (w505:sgl[])
                      n196 = To Variant(anything=w504) -> (Variant=w529:variant)
                      n197 = To Variant(anything=w505) -> (Variant=w531:variant)
                      n198 = invoke class="INanoScanII" method="NsAsReadProfile"(reference=w534, error in=w533, "sAperture"=w532, "fStartPosition"=w528, "fEndPosition"=w527, "sDecimationFactor"=i16 100, "pvarProfileAmplitude"=w531, "pvarProfilePosition"=w529) -> (reference out=w523:refnum<k7>, error out=w524:errorcluster, "sAperture"=w521:i16, "pvarProfileAmplitude"=w526:variant, "pvarProfilePosition"=w525:variant)  [unwired: 1 in, 4 out]
                      n199 = Variant To Data(error in=w524, type=w503, Variant=w526) -> (data=w502:sgl[])  [unwired: 1 out]
                      n200 = Variant To Data(error in=w524, type=w503, Variant=w525) -> (data=w501:sgl[], error out=w522:errorcluster)
                      n201 = local write "Intensity"(w502) -> ()
                      n202 = local write "Position"(w501) -> ()
                      n203 = Bundle("Intensity"=w501, "Intensity"=w502) -> (→"Aperture 2":cluster{"Intensity":sgl[], "Intensity":sgl[]})  [unwired: 1 out]
                      n204 = invoke class="INanoScanII" method="NsAsGetNumberOfROIs"(reference=w523, error in=w522, "sAperture"=w521, "psNumberOfROIs"="ROIs Ap2") -> (reference out=w520:refnum<k7>, error out=w519:errorcluster, "sAperture"=w518:i16, "psNumberOfROIs"=w512:i16)  [unwired: 1 in, 1 out]
                      n205 = local read "Sampling Res 2"() -> (w513:sgl)
                      n206 = invoke class="INanoScanII" method="NsAsGetSamplingResolution"(reference=w520, error in=w519, "sAperture"=w518, "pfSamplingResolution"=w513) -> (reference out=w517:refnum<k7>, error out=w516:errorcluster, "sAperture"=w515:i16, "pfSamplingResolution"=w514:sgl)  [unwired: 1 in, 1 out]
                      n207 = local write "Sampling Res 2"(w514) -> ()
                      n208 = local read "Gain2"() -> (w507:u32)
                      n209 = invoke class="INanoScanII" method="NsAsGetGain"(reference=w517, error in=w516, "sAperture"=w515, "psGain"=w507) -> (reference out=w510:refnum<k7>, error out=w511:errorcluster, "psGain"=→"Gain2":i16)  [unwired: 1 in, 2 out]
                      n210 = for {
                        N: w512 -> [_]
                        tunnel: w541 -> [w551]
                        tunnel: w540 -> [w548]
                        tunnel: [TRUE] -> w498 mode=indexing
                        tunnel: w511 -> [w546]
                        tunnel: w510 -> [w542]
                        tunnel: [w545] -> w509
                        tunnel: [w544] -> w508
                        i -> [w543]
                        n211 = Number To Boolean Array(number=w551) -> (Boolean array=w549:bool[])
                        n212 = Array Size(array=w549) -> (size(s)=w550:i32)
                        n213 = for {
                          N: w550 -> [_]
                          tunnel: w549 -> [w554]
                          tunnel: w548 -> [w560]
                          tunnel: w543 -> [w559]
                          tunnel: w546 -> [w558]
                          tunnel: w542 -> [w557]
                          tunnel: [w556] -> w545
                          tunnel: [w555] -> w544
                          i -> [w553]
                          n214 = Index Array(array=w554, index=w553) -> (element=w552:bool)
                          n215 = case shown="10" w553 {
                            tunnel: w552 -> [w568 w597 _ w628 w659 w688 w717 w744 w775 w804 w841]
                            tunnel: w560 -> [w567 w595 _ w629 w655 w687 w716 w746 w774 w803 w840]
                            tunnel: w559 -> [w566 w590 _ w627 w654 w686 w715 w745 w773 w802 w839]
                            tunnel: w553 -> [w565 w596 _ w630 _ _ _ _ _ _ _]
                            tunnel: w558 -> [w564 w593 w621 w625 w653 w683 w713 w742 w771 w798 w835]
                            tunnel: w557 -> [w563 w594 w622 w626 w658 w682 w714 w743 w772 w799 w836]
                            tunnel: [w562 w591 w622 w624 w657 w685 w712 w741 w770 w801 w838] -> w556
                            tunnel: [w561 w592 w621 w623 w656 w684 w711 w740 w769 w800 w837] -> w555
                            frame 0 {
                              n216 = case shown="True" w568 {
                                tunnel: w567 -> [_ w574]
                                tunnel: w566 -> [_ w573]
                                tunnel: w565 -> [_ _]
                                tunnel: w564 -> [w569 w579]
                                tunnel: w563 -> [w570 w578]
                                tunnel: [w570 w577] -> w562
                                tunnel: [w569 w576] -> w561
                                frame False {
                                }
                                frame True {
                                n217 = local read "BeamWidth"() -> (w571:sgl)
                                n218 = invoke class="INanoScanII" method="NsAsGetBeamWidth"(reference=w578, error in=w579, "sAperture"=w574, "sROIIndex"=w573, "fClipLevel"=13.5, "pfBeamWidth"=w571) -> (reference out=w577:refnum<k7>, error out=w576:errorcluster, "pfBeamWidth"=w572:sgl)  [unwired: 1 in, 4 out]
                                n219 = Number To Decimal String(number=w574) -> (decimal integer string=w588:string)  [unwired: 1 out]
                                n220 = Number To Fractional String(number=w572, precision (6)=i16 2) -> (F-format string=w586:string)  [unwired: 2 out]
                                n221 = Number To Decimal String(number=w573) -> (decimal integer string=w587:string)  [unwired: 1 out]
                                n222 = Build Array("13.5% Width", w588, w587, w586) -> (w585:string[])
                                n223 = local read "Row"() -> (w581:i32)
                                n224 = local read "Parameters Array"() -> (w583:string[][])
                                n225 = Insert Into Array(array=w583, index (row)=w581, new element=w585) -> (w582:string[][])  [unwired: 1 in]
                                n226 = local write "Parameters Array"(w582) -> ()
                                n227 = Increment(x=w581) -> (x+1=w584:i32)
                                n228 = local write "Row"(w584) -> ()
                                }
                              }
                            }
                            frame 1 {
                              n229 = case shown="True" w597 {
                                tunnel: w596 -> [_ _]
                                tunnel: w595 -> [_ w608]
                                tunnel: w594 -> [w598 w610]
                                tunnel: w593 -> [w599 w609]
                                tunnel: [w599 w600] -> w592
                                tunnel: [w598 w602] -> w591
                                tunnel: w590 -> [_ w607]
                                frame False {
                                }
                                frame True {
                                n230 = local read "BeamWidth"() -> (w605:sgl)
                                n231 = invoke class="INanoScanII" method="NsAsGetBeamWidth"(reference=w610, error in=w609, "sAperture"=w608, "sROIIndex"=w607, "fClipLevel"=sgl 50.0, "pfBeamWidth"=w605) -> (reference out=w602:refnum<k7>, error out=w600:errorcluster, "sAperture"=w601:i16, "sROIIndex"=w604:i16, "pfBeamWidth"=w603:sgl)  [unwired: 1 in, 2 out]
                                n232 = Number To Decimal String(number=w601) -> (decimal integer string=w619:string)  [unwired: 1 out]
                                n233 = Number To Decimal String(number=w604) -> (decimal integer string=w618:string)  [unwired: 1 out]
                                n234 = Number To Fractional String(number=w603, precision (6)=i16 2) -> (F-format string=w617:string)  [unwired: 2 out]
                                n235 = Build Array("50.0% Width", w619, w618, w617) -> (w615:string[])
                                n236 = local read "Row"() -> (w613:i32)
                                n237 = local read "Parameters Array"() -> (w616:string[][])
                                n238 = Increment(x=w613) -> (x+1=w612:i32)
                                n239 = Insert Into Array(array=w616, index (row)=w613, new element=w615) -> (w614:string[][])  [unwired: 1 in]
                                n240 = local write "Row"(w612) -> ()
                                n241 = local write "Parameters Array"(w614) -> ()
                                }
                              }
                            }
                            frame Default {
                            }
                            frame 4 {
                              n242 = case shown="True" w628 {
                                tunnel: w630 -> [_ _]
                                tunnel: w629 -> [_ w637]
                                tunnel: w627 -> [_ w636]
                                tunnel: w626 -> [w632 w642]
                                tunnel: w625 -> [w631 w641]
                                tunnel: [w632 w640] -> w624
                                tunnel: [w631 w639] -> w623
                                frame False {
                                }
                                frame True {
                                n243 = local read "BeamWidth"() -> (w638:sgl)
                                n244 = invoke class="INanoScanII" method="NsAsGetBeamWidth4Sigma"(reference=w642, error in=w641, "sAperture"=w637, "sROIIndex"=w636, "pfBeamWidth4Sigma"=w638) -> (reference out=w640:refnum<k7>, error out=w639:errorcluster, "sAperture"=w635:i16, "sROIIndex"=w634:i16, "pfBeamWidth4Sigma"=w633:sgl)  [unwired: 1 in, 1 out]
                                n245 = Number To Decimal String(number=w635) -> (decimal integer string=w651:string)  [unwired: 1 out]
                                n246 = Number To Decimal String(number=w634) -> (decimal integer string=w650:string)  [unwired: 1 out]
                                n247 = Number To Fractional String(number=w633, precision (6)=i16 2) -> (F-format string=w649:string)  [unwired: 2 out]
                                n248 = Build Array("4Sigma Width", w651, w650, w649) -> (w648:string[])
                                n249 = local read "Row"() -> (w645:i32)
                                n250 = local read "Parameters Array"() -> (w646:string[][])
                                n251 = Insert Into Array(array=w646, index (row)=w645, new element=w648) -> (w647:string[][])  [unwired: 1 in]
                                n252 = Increment(x=w645) -> (x+1=w644:i32)
                                n253 = local write "Parameters Array"(w647) -> ()
                                n254 = local write "Row"(w644) -> ()
                                }
                              }
                            }
                            frame 5 {
                              n255 = case shown="True" w659 {
                                tunnel: w658 -> [w660 w671]
                                tunnel: [w660 w670] -> w657
                                tunnel: [w661 w669] -> w656
                                tunnel: w655 -> [_ w668]
                                tunnel: w654 -> [_ w667]
                                tunnel: w653 -> [w661 w663]
                                frame False {
                                }
                                frame True {
                                n256 = local read "Centroid Pos"() -> (w662:sgl)
                                n257 = invoke class="INanoScanII" method="NsAsGetCentroidPosition"(reference=w671, error in=w663, "sAperture"=w668, "sROIIndex"=w667, "pfCentroidPosition"=w662) -> (reference out=w670:refnum<k7>, error out=w669:errorcluster, "sAperture"=w666:i16, "sROIIndex"=w665:i16, "pfCentroidPosition"=w664:sgl)  [unwired: 1 in, 1 out]
                                n258 = Number To Decimal String(number=w666) -> (decimal integer string=w680:string)  [unwired: 1 out]
                                n259 = Number To Decimal String(number=w665) -> (decimal integer string=w679:string)  [unwired: 1 out]
                                n260 = Number To Fractional String(number=w664, precision (6)=i16 2) -> (F-format string=w678:string)  [unwired: 2 out]
                                n261 = Build Array("Centroid Position", w680, w679, w678) -> (w677:string[])
                                n262 = local read "Row"() -> (w673:i32)
                                n263 = local read "Parameters Array"() -> (w676:string[][])
                                n264 = Increment(x=w673) -> (x+1=w674:i32)
                                n265 = Insert Into Array(array=w676, index (row)=w673, new element=w677) -> (w675:string[][])  [unwired: 1 in]
                                n266 = local write "Parameters Array"(w675) -> ()
                                n267 = local write "Row"(w674) -> ()
                                }
                              }
                            }
                            frame 6 {
                              n268 = case shown="True" w688 {
                                tunnel: w687 -> [_ w695]
                                tunnel: w686 -> [_ w694]
                                tunnel: [w690 w700] -> w685
                                tunnel: [w689 w699] -> w684
                                tunnel: w683 -> [w689 w698]
                                tunnel: w682 -> [w690 w697]
                                frame False {
                                }
                                frame True {
                                n269 = local read "Peak"() -> (w696:sgl)
                                n270 = invoke class="INanoScanII" method="NsAsGetPeakPosition"(reference=w697, error in=w698, "sAperture"=w695, "sROIIndex"=w694, "pfPeakPosition"=w696) -> (reference out=w700:refnum<k7>, error out=w699:errorcluster, "sAperture"=w693:i16, "sROIIndex"=w692:i16, "pfPeakPosition"=w691:sgl)  [unwired: 1 in, 1 out]
                                n271 = Number To Decimal String(number=w693) -> (decimal integer string=w709:string)  [unwired: 1 out]
                                n272 = Number To Decimal String(number=w692) -> (decimal integer string=w708:string)  [unwired: 1 out]
                                n273 = Number To Fractional String(number=w691, precision (6)=i16 2) -> (F-format string=w707:string)  [unwired: 2 out]
                                n274 = Build Array("Peak Position", w709, w708, w707) -> (w706:string[])
                                n275 = local read "Row"() -> (w703:i32)
                                n276 = local read "Parameters Array"() -> (w704:string[][])
                                n277 = Increment(x=w703) -> (x+1=w702:i32)
                                n278 = Insert Into Array(array=w704, index (row)=w703, new element=w706) -> (w705:string[][])  [unwired: 1 in]
                                n279 = local write "Row"(w702) -> ()
                                n280 = local write "Parameters Array"(w705) -> ()
                                }
                              }
                            }
                            frame 7 {
                              n281 = case shown="True" w717 {
                                tunnel: w716 -> [_ w727]
                                tunnel: w715 -> [_ w726]
                                tunnel: w714 -> [w719 w729]
                                tunnel: w713 -> [w718 w728]
                                tunnel: [w719 w725] -> w712
                                tunnel: [w718 w724] -> w711
                                frame False {
                                }
                                frame True {
                                n282 = local read "Centroid Pos"() -> (w720:sgl)
                                n283 = invoke class="INanoScanII" method="NsAsGetCentroidSeparation"(reference=w729, error in=w728, "sAperture"=w727, "sROIIndex"=w726, "pfCentroidSeparation"=w720) -> (reference out=w725:refnum<k7>, error out=w724:errorcluster, "sAperture"=w723:i16, "sROIIndex"=w722:i16, "pfCentroidSeparation"=w721:sgl)  [unwired: 1 in, 1 out]
                                n284 = Number To Decimal String(number=w723) -> (decimal integer string=w738:string)  [unwired: 1 out]
                                n285 = Number To Decimal String(number=w722) -> (decimal integer string=w737:string)  [unwired: 1 out]
                                n286 = Number To Fractional String(number=w721, precision (6)=i16 2) -> (F-format string=w736:string)  [unwired: 2 out]
                                n287 = Build Array("Centroid Separation", w738, w737, w736) -> (w733:string[])
                                n288 = local read "Row"() -> (w732:i32)
                                n289 = local read "Parameters Array"() -> (w735:string[][])
                                n290 = Insert Into Array(array=w735, index (row)=w732, new element=w733) -> (w734:string[][])  [unwired: 1 in]
                                n291 = Increment(x=w732) -> (x+1=w731:i32)
                                n292 = local write "Row"(w731) -> ()
                                n293 = local write "Parameters Array"(w734) -> ()
                                }
                              }
                            }
                            frame 8 {
                              n294 = case shown="True" w744 {
                                tunnel: w746 -> [_ w751]
                                tunnel: w745 -> [_ w750]
                                tunnel: w743 -> [w748 w758]
                                tunnel: w742 -> [w747 w757]
                                tunnel: [w748 w756] -> w741
                                tunnel: [w747 w755] -> w740
                                frame False {
                                }
                                frame True {
                                n295 = local read "Peak"() -> (w749:sgl)
                                n296 = invoke class="INanoScanII" method="NsAsGetPeakSeparation"(reference=w758, error in=w757, "sAperture"=w751, "sROIIndex"=w750, "pfPeakSeparation"=w749) -> (reference out=w756:refnum<k7>, error out=w755:errorcluster, "sAperture"=w754:i16, "sROIIndex"=w753:i16, "pfPeakSeparation"=w752:sgl)  [unwired: 1 in, 1 out]
                                n297 = Number To Decimal String(number=w754) -> (decimal integer string=w767:string)  [unwired: 1 out]
                                n298 = Number To Decimal String(number=w753) -> (decimal integer string=w766:string)  [unwired: 1 out]
                                n299 = Number To Fractional String(number=w752, precision (6)=i16 2) -> (F-format string=w765:string)  [unwired: 2 out]
                                n300 = Build Array("Peak Separation", w767, w766, w765) -> (w762:string[])
                                n301 = local read "Row"() -> (w761:i32)
                                n302 = local read "Parameters Array"() -> (w764:string[][])
                                n303 = Insert Into Array(array=w764, index (row)=w761, new element=w762) -> (w763:string[][])  [unwired: 1 in]
                                n304 = Increment(x=w761) -> (x+1=w760:i32)
                                n305 = local write "Parameters Array"(w763) -> ()
                                n306 = local write "Row"(w760) -> ()
                                }
                              }
                            }
                            frame 9 {
                              n307 = case shown="True" w775 {
                                tunnel: w774 -> [_ w784]
                                tunnel: w773 -> [_ w783]
                                tunnel: w772 -> [w777 w787]
                                tunnel: w771 -> [w776 w786]
                                tunnel: [w777 w785] -> w770
                                tunnel: [w776 w779] -> w769
                                frame False {
                                }
                                frame True {
                                n308 = local read "Irradiance"() -> (w778:sgl)
                                n309 = invoke class="INanoScanII" method="NsAsGetBeamIrradiance"(reference=w787, error in=w786, "sAperture"=w784, "sROIIndex"=w783, "pfBeamIrradiance"=w778) -> (reference out=w785:refnum<k7>, error out=w779:errorcluster, "sAperture"=w782:i16, "sROIIndex"=w781:i16, "pfBeamIrradiance"=w780:sgl)  [unwired: 1 in, 1 out]
                                n310 = Number To Decimal String(number=w782) -> (decimal integer string=w796:string)  [unwired: 1 out]
                                n311 = Number To Decimal String(number=w781) -> (decimal integer string=w795:string)  [unwired: 1 out]
                                n312 = Number To Fractional String(number=w780, precision (6)=i16 2) -> (F-format string=w794:string)  [unwired: 2 out]
                                n313 = Build Array("Irradiance", w796, w795, w794) -> (w791:string[])
                                n314 = local read "Parameters Array"() -> (w793:string[][])
                                n315 = local read "Row"() -> (w790:i32)
                                n316 = Insert Into Array(array=w793, index (row)=w790, new element=w791) -> (w792:string[][])  [unwired: 1 in]
                                n317 = Increment(x=w790) -> (x+1=w789:i32)
                                n318 = local write "Parameters Array"(w792) -> ()
                                n319 = local write "Row"(w789) -> ()
                                }
                              }
                            }
                            frame 10 {
                              n320 = case shown="True" w804 {
                                tunnel: w803 -> [_ w816]
                                tunnel: w802 -> [_ w815]
                                tunnel: [w806 w818] -> w801
                                tunnel: [w805 w817] -> w800
                                tunnel: w799 -> [w806 w810]
                                tunnel: w798 -> [w805 w809]
                                frame False {
                                }
                                frame True {
                                n321 = local read "Goodness"() -> (w807:sgl)
                                n322 = local read "Roughness"() -> (w808:sgl)
                                n323 = invoke class="INanoScanII" method="NsAsGetGaussianFit"(reference=w810, error in=w809, "sAperture"=w816, "sROIIndex"=w815, "pfGoodnessFit"=w807, "pfRoughnessFit"=w808) -> (reference out=w818:refnum<k7>, error out=w817:errorcluster, "sAperture"=w814:i16, "sROIIndex"=w813:i16, "pfGoodnessFit"=w812:sgl, "pfRoughnessFit"=w811:sgl)  [unwired: 1 in, 1 out]
                                n324 = Number To Decimal String(number=w814) -> (decimal integer string=w831:string)  [unwired: 1 out]
                                n325 = Number To Decimal String(number=w813) -> (decimal integer string=w830:string)  [unwired: 1 out]
                                n326 = Number To Fractional String(number=w812, precision (6)=i16 2) -> (F-format string=w833:string)  [unwired: 2 out]
                                n327 = Number To Fractional String(number=w811, precision (6)=i16 2) -> (F-format string=w829:string)  [unwired: 2 out]
                                n328 = local read "Row"() -> (w824:i32)
                                n329 = Build Array("Goodness of Fit", w831, w830, w833) -> (w828:string[])
                                n330 = Build Array("Roughness of Fit", w831, w830, w829) -> (w827:string[])
                                n331 = local read "Parameters Array"() -> (w821:string[][])
                                n332 = Insert Into Array(array=w821, index (row)=w824, new element=w828) -> (w826:string[][])  [unwired: 1 in]
                                n333 = Increment(x=w824) -> (x+1=w823:i32)
                                n334 = local write "Parameters Array"(w826) -> ()
                                n335 = Insert Into Array(array=w826, index (row)=w823, new element=w827) -> (w825:string[][])  [unwired: 1 in]
                                n336 = Increment(x=w823) -> (x+1=w822:i32)
                                n337 = local write "Parameters Array"(w825) -> ()
                                n338 = local write "Row"(w822) -> ()
                                }
                              }
                            }
                            frame 11 {
                              n339 = case shown="True" w841 {
                                tunnel: w840 -> [_ _]
                                tunnel: w839 -> [_ w847]
                                tunnel: [w843 w851] -> w838
                                tunnel: [w842 w850] -> w837
                                tunnel: w836 -> [w843 w849]
                                tunnel: w835 -> [w842 w848]
                                frame False {
                                }
                                frame True {
                                n340 = local read "Ellipticity"() -> (w844:sgl)
                                n341 = invoke class="INanoScanII" method="NsAsGetBeamEllipticity"(reference=w849, error in=w848, "sROIIndex"=w847, "pfBeamEllipticity"=w844) -> (reference out=w851:refnum<k7>, error out=w850:errorcluster, "sROIIndex"=w846:i16, "pfBeamEllipticity"=w845:sgl)  [unwired: 1 in, 1 out]
                                n342 = Number To Decimal String(number=w846) -> (decimal integer string=w859:string)  [unwired: 1 out]
                                n343 = Number To Fractional String(number=w845, precision (6)=i16 2) -> (F-format string=w858:string)  [unwired: 2 out]
                                n344 = Build Array("Ellipticity", "", w859, w858) -> (w855:string[])
                                n345 = local read "Row"() -> (w854:i32)
                                n346 = local read "Parameters Array"() -> (w857:string[][])
                                n347 = Insert Into Array(array=w857, index (row)=w854, new element=w855) -> (w856:string[][])  [unwired: 1 in]
                                n348 = Increment(x=w854) -> (x+1=w853:i32)
                                n349 = local write "Parameters Array"(w856) -> ()
                                n350 = local write "Row"(w853) -> ()
                                }
                              }
                            }
                          }
                        }
                      }
                      "ROIs Aperture 2" <- w498
                    }
                  }
                }
                n351 = stacked-sequence {
                  tunnel: w106 -> [_ w121]
                  tunnel: [_ w121] -> w104
                  frame #0 {
                    n352 = local read "Parameters Array"() -> (w120:string[][])
                    n353 = property on="Parameters" class="MCListbox (strict)"("Item Names"=w120) -> ()  [unwired: 2 in, 2 out]
                  }
                  frame #1 {
                    n354 = Initialize Array("", 1, 4) -> (→"Parameters Array":string[][])
                    n355 = local write "Row"(0) -> ()
                  }
                }
              }
            }
            n356 = case shown="0" w95 {
              tunnel: w72 -> [_ w952 _ _ _ _]
              tunnel: w70 -> [w872 w950 w964 w974 w987 w997]
              tunnel: w71 -> [w871 w951 w963 w973 w988 w998]
              tunnel: [w870 w949 w962 w972 w986 w998] -> w69
              tunnel: [w869 w948 w961 w971 w985 w997] -> w68
              frame 0 {
                # "Do an AutoFind\nGet the profiles"
                n357 = stacked-sequence {
                  tunnel: w871 -> [w878 _]
                  tunnel: w872 -> [w877 _]
                  tunnel: [w874 _] -> w870
                  tunnel: [w873 _] -> w869
                  frame #0 {
                    n358 = invoke class="INanoScanII" method="NsAsAutoFind"(reference=w878, error in=w877) -> (reference out=w876:refnum<k7>, error out=w875:errorcluster)  [unwired: 1 in, 1 out]
                    n359 = for {
                      N: 2 -> [_]
                      tunnel: w876 -> [w884]
                      tunnel: w875 -> [w883]
                      tunnel: [w881] -> w874
                      tunnel: [w880] -> w873
                      i -> [w882]
                      n360 = case shown="0, Default" w882 {
                        tunnel: w884 -> [w910 w941]
                        tunnel: w883 -> [w909 w940]
                        tunnel: w882 -> [w908 w939]
                        tunnel: [w886 w917] -> w881
                        tunnel: [w885 w916] -> w880
                        frame 0, Default {
                          w895 = sgl[] [] ("Intensity")
                          n361 = local read "AprLeft"() -> (w907:sgl)
                          n362 = local read "Intensity"() -> (w911:sgl[])
                          n363 = local read "Apr Right"() -> (w906:sgl)
                          n364 = invoke class="INanoScanII" method="NsAsGetApertureLimits"(reference=w910, error in=w909, "sAperture"=w908, "pfLeftBound"=w907, "pfRightBound"=w906) -> (reference out=w905:refnum<k7>, error out=w904:errorcluster, "sAperture"=w903:i16, "pfLeftBound"=w902:sgl, "pfRightBound"=w901:sgl)  [unwired: 1 in, 1 out]
                          n365 = To Variant(anything=w911) -> (Variant=w899:variant)
                          n366 = local read "Position"() -> (w912:sgl[])
                          n367 = To Variant(anything=w912) -> (Variant=w898:variant)
                          n368 = invoke class="INanoScanII" method="NsAsReadProfile"(reference=w905, error in=w904, "sAperture"=w903, "fStartPosition"=w902, "fEndPosition"=w901, "sDecimationFactor"=i16 100, "pvarProfileAmplitude"=w899, "pvarProfilePosition"=w898) -> (reference out=w891:refnum<k7>, error out=w894:errorcluster, "sAperture"=w889:i16, "pvarProfileAmplitude"=w897:variant, "pvarProfilePosition"=w896:variant)  [unwired: 1 in, 4 out]
                          n369 = Variant To Data(error in=w894, type=w895, Variant=w897) -> (data=w893:sgl[])  [unwired: 1 out]
                          n370 = Variant To Data(error in=w894, type=w895, Variant=w896) -> (data=w892:sgl[], error out=w890:errorcluster)
                          n371 = local write "Intensity"(w893) -> ()
                          n372 = local write "Position"(w892) -> ()
                          n373 = Bundle("Intensity"=w892, "Intensity"=w893) -> (w914:cluster{"Intensity":sgl[], "Intensity":sgl[]})  [unwired: 1 out]
                          n374 = local write "Aperture 1"(w914) -> ()
                          n375 = local read "ROIs AP1"() -> (w888:i16)
                          n376 = invoke class="INanoScanII" method="NsAsGetNumberOfROIs"(reference=w891, error in=w890, "sAperture"=w889, "psNumberOfROIs"=w888) -> (reference out=w886:refnum<k7>, error out=w885:errorcluster, "psNumberOfROIs"=w887:i16)  [unwired: 1 in, 2 out]
                          n377 = for {
                            N: w887 -> [_]
                            tunnel: [TRUE] -> w913 mode=indexing
                          }
                          n378 = local write "ROIs Aperture1"(w913) -> ()
                        }
                        frame 1 {
                          w926 = sgl[] [] ("Intensity")
                          n379 = local read "AprLeft"() -> (w938:sgl)
                          n380 = local read "Intensity"() -> (w942:sgl[])
                          n381 = local read "Apr Right"() -> (w937:sgl)
                          n382 = invoke class="INanoScanII" method="NsAsGetApertureLimits"(reference=w941, error in=w940, "sAperture"=w939, "pfLeftBound"=w938, "pfRightBound"=w937) -> (reference out=w936:refnum<k7>, error out=w935:errorcluster, "sAperture"=w934:i16, "pfLeftBound"=w933:sgl, "pfRightBound"=w932:sgl)  [unwired: 1 in, 1 out]
                          n383 = To Variant(anything=w942) -> (Variant=w930:variant)
                          n384 = local read "Position"() -> (w943:sgl[])
                          n385 = To Variant(anything=w943) -> (Variant=w929:variant)
                          n386 = invoke class="INanoScanII" method="NsAsReadProfile"(reference=w936, error in=w935, "sAperture"=w934, "fStartPosition"=w933, "fEndPosition"=w932, "sDecimationFactor"=i16 100, "pvarProfileAmplitude"=w930, "pvarProfilePosition"=w929) -> (reference out=w922:refnum<k7>, error out=w925:errorcluster, "sAperture"=w920:i16, "pvarProfileAmplitude"=w928:variant, "pvarProfilePosition"=w927:variant)  [unwired: 1 in, 4 out]
                          n387 = Variant To Data(error in=w925, type=w926, Variant=w928) -> (data=w924:sgl[])  [unwired: 1 out]
                          n388 = Variant To Data(error in=w925, type=w926, Variant=w927) -> (data=w923:sgl[], error out=w921:errorcluster)
                          n389 = local write "Intensity"(w924) -> ()
                          n390 = local write "Position"(w923) -> ()
                          n391 = Bundle("Intensity"=w923, "Intensity"=w924) -> (w945:cluster{"Intensity":sgl[], "Intensity":sgl[]})  [unwired: 1 out]
                          n392 = local write "Aperture 2"(w945) -> ()
                          n393 = local read "ROIs Ap2"() -> (w919:i16)
                          n394 = invoke class="INanoScanII" method="NsAsGetNumberOfROIs"(reference=w922, error in=w921, "sAperture"=w920, "psNumberOfROIs"=w919) -> (reference out=w917:refnum<k7>, error out=w916:errorcluster, "psNumberOfROIs"=w918:i16)  [unwired: 1 in, 2 out]
                          n395 = for {
                            N: w918 -> [_]
                            tunnel: [TRUE] -> w944 mode=indexing
                          }
                          n396 = local write "ROIs Aperture 2"(w944) -> ()
                        }
                      }
                    }
                  }
                  frame #1 {
                    w947 = FALSE
                    n397 = local write "Auto Find"(w947) -> ()
                    n398 = local write "Boolean"(w947) -> ()
                  }
                }
              }
              frame 1 {
                # "Set the Rotation Rate"
                n399 = stacked-sequence {
                  tunnel: w952 -> [w959 _]
                  tunnel: w951 -> [w956 _]
                  tunnel: w950 -> [w957 _]
                  tunnel: [w954 _] -> w949
                  tunnel: [w953 _] -> w948
                  frame #0 {
                    n400 = Index Array(array=w959, index="Select Rotation Rate") -> (element=w955:sgl)
                    n401 = invoke class="INanoScanII" method="NsAsSetRotationFrequency"(reference=w956, error in=w957, "fRotationFrequency"=w955) -> (reference out=w954:refnum<k7>, error out=w953:errorcluster)  [unwired: 1 in, 2 out]
                  }
                  frame #1 {
                    w960 = FALSE
                    n402 = local write "Set Rotation"(w960) -> ()
                    n403 = local write "Boolean"(w960) -> ()
                  }
                }
              }
              frame 2 {
                # "Set the sampling rate"
                n404 = stacked-sequence {
                  tunnel: w964 -> [w968 _]
                  tunnel: w963 -> [w969 _]
                  tunnel: [w966 _] -> w962
                  tunnel: [w965 _] -> w961
                  frame #0 {
                    n405 = invoke class="INanoScanII" method="NsAsSetSamplingResolution"(reference=w969, error in=w968, "fSamplingResolution"="Select Sampling") -> (reference out=w966:refnum<k7>, error out=w965:errorcluster)  [unwired: 1 in, 2 out]
                  }
                  frame #1 {
                    w970 = FALSE
                    n406 = local write "Set Sampling"(w970) -> ()
                    n407 = local write "Boolean"(w970) -> ()
                  }
                }
              }
              frame 3 {
                # "Set the gain for the selected aperture"
                n408 = stacked-sequence {
                  tunnel: w974 -> [w979 _]
                  tunnel: w973 -> [w980 _]
                  tunnel: [w976 _] -> w972
                  tunnel: [w975 _] -> w971
                  frame #0 {
                    n409 = local read "Gains"() -> (w982:u32[])
                    n410 = Decrement(x="Aperture") -> (x-1=w977:i32)
                    n411 = Index Array(array=w982, index="Gain") -> (element=w978:u32)
                    n412 = invoke class="INanoScanII" method="NsAsSetGain"(reference=w980, error in=w979, "sAperture"=w977, "sGain"=w978) -> (reference out=w976:refnum<k7>, error out=w975:errorcluster)  [unwired: 1 in, 3 out]
                  }
                  frame #1 {
                    w984 = FALSE
                    n413 = local write "Boolean"(w984) -> ()
                    n414 = local write "Set Gain"(w984) -> ()
                  }
                }
              }
              frame 4 {
                # "Set the filter for the selected Aperture"
                n415 = stacked-sequence {
                  tunnel: w988 -> [w994 _]
                  tunnel: w987 -> [w993 _]
                  tunnel: [w990 _] -> w986
                  tunnel: [w989 _] -> w985
                  frame #0 {
                    n416 = local read "Aperture"() -> (w995:i32)
                    n417 = Decrement(x=w995) -> (x-1=w992:i32)
                    n418 = invoke class="INanoScanII" method="NsAsSetFilter"(reference=w994, error in=w993, "sAperture"=w992, "fFilter"="Filter") -> (reference out=w990:refnum<k7>, error out=w989:errorcluster)  [unwired: 1 in, 3 out]
                  }
                  frame #1 {
                    w996 = FALSE
                    n419 = local write "Set Filter"(w996) -> ()
                    n420 = local write "Boolean"(w996) -> ()
                  }
                }
              }
              frame Default {
              }
            }
          }
        }
      }
      n421 = Close Reference(reference=w9, error in (no error)=w8) -> (error out=w7:errorcluster)
    }
    frame True {
      n422 = Not(x=w1002) -> (.not. x?=w1001:bool)
      n423 = local write "Boolean"(w1001) -> ()
      n424 = Close Reference(reference=w999) -> ()  [unwired: 1 in, 1 out]
      n425 = One Button Dialog(message="Cannot open NanoScan Automation Server") -> ()  [unwired: 2 out]
    }
  }
  "error out" <- w2
  "Boolean" <- w1
